vi "Fetch Measurement.vi"(8 "error in (no error)":errorcluster, 9 "Timeout (10000 ms)":u32=10000, 11 "VISA resource name":refnum<visa-resource-name>) -> (0 "error out":errorcluster, 1 "End of Data?":bool, 2 "Measurements":dbl[](array[numeric]), 3 "VISA resource name out":refnum<visa-resource-name>)   [LabVIEW 2020, in "Agilent 34401.lvlib"]
doc: "Fetches the measurement according to the instrument model, trigger source, and math configuration.\n\n<B>Note:</B>\n\nThis VI does not check the instrument status. Typically, you call this VI only in a sequence of calls to other low-level instrument driver VIs. The sequence performs one operation. You use the low-level VIs to optimize one or more aspects of interaction with the instrument. If you want to check the instrument status, call the <B>Error Query VI</B> at the conclusion of the sequence."
uses:
  Agilent 34401.lvlib
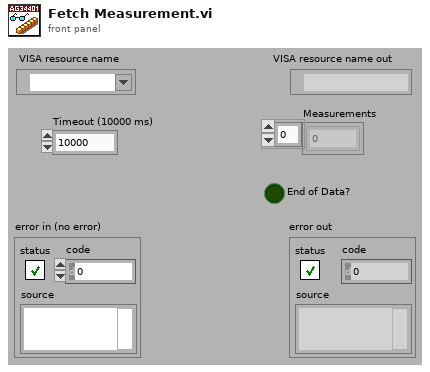
[diagram p1: front panel]
types:
  T1 = typedef "Agilent 34401.lvlib/Extended User Data.ctl" = cluster{"Trigger Source":u16, "Math Storage":u16, "Agilent Model":i32}
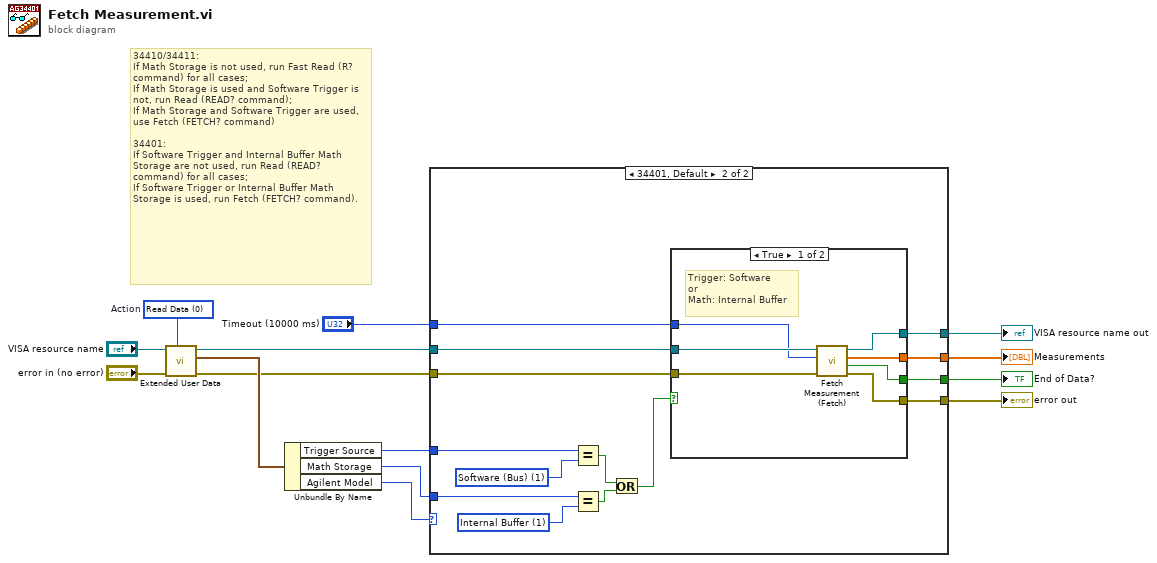
[diagram p0: block diagram]
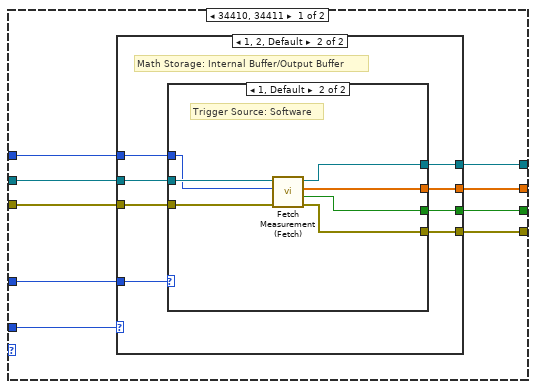
[diagram p2: hidden frame]
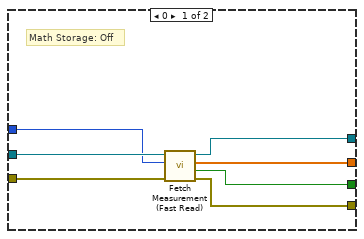
[diagram p3: hidden frame]
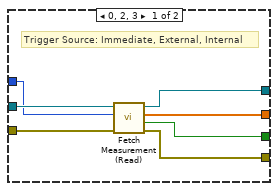
[diagram p4: hidden frame]
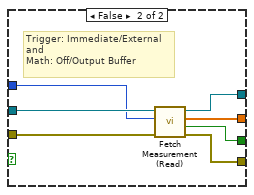
[diagram p5: hidden frame]
diagram:
  w12 = u16 0 items=["Read Data", "Write Data", "Dispose of Data"]  # Action
  # "34410/34411:\nIf Math Storage is not used, run Fast Read (R? command) for all cases;\nIf Math Storage is used and Software Trigger is not, run Read (READ? command);\nIf Math Storage and Software Trigger are used, use Fetch (FETCH? command)\n\n34401:\nIf Software Trigger and Internal Buffer Math Storage are not used, run Read (READ? command) for all cases;\nIf Software Trigger or Internal Buffer Math Storage is used, run Fetch (FETCH? command)."
  n1 = call "Extended User Data.vi"("Action (0: Read Data)"=w12, "Error In (no error)"="error in (no error)", "VISA resource name in"="VISA resource name") -> ("Error Out"=w6:errorcluster, "User Data Out"=w11:T1, "VISA resource name out"=w5:refnum<visa-resource-name>)  [unwired: 6 in]
  n2 = Unbundle By Name(w11) -> ("Trigger Source"=w10:u16, "Math Storage"=w9:u16, "Agilent Model"=w8:i32)
  n3 = case shown="34401, Default" w8 {
    tunnel: w9 -> [w20 w64]
    tunnel: w10 -> [w15 w63]
    tunnel: "Timeout (10000 ms)" -> [w23 w60]
    tunnel: w6 -> [w21 w62]
    tunnel: w5 -> [w22 w61]
    tunnel: [w18 w57] -> w4
    tunnel: [w16 w58] -> w3
    tunnel: [w17 w59] -> w2
    tunnel: [w19 w56] -> w1
    frame 34410, 34411 {
      n4 = case shown="1, 2, Default" w20 {
        tunnel: w23 -> [w28 w35]
        tunnel: w22 -> [w30 w36]
        tunnel: w21 -> [w29 w37]
        tunnel: [w27 w34] -> w19
        tunnel: [w26 w33] -> w18
        tunnel: [w25 w32] -> w17
        tunnel: [w24 w31] -> w16
        tunnel: w15 -> [_ w38]
        frame 0 {
          # "Math Storage: Off"
          n5 = call "Fetch Measurement (Fast Read).vi"("error in (no error)"=w29, "Timeout (10000 ms)"=w28, "VISA resource name"=w30) -> ("error out"=w25:errorcluster, "End of Data?"=w24:bool, "Measurements"=w26:dbl[], "VISA resource name out"=w27:refnum<visa-resource-name>)  [unwired: 5 in]
        }
        frame 1, 2, Default {
          # "Math Storage: Internal Buffer/Output Buffer"
          n6 = case shown="1, Default" w38 {
            tunnel: w37 -> [w44 w52]
            tunnel: w36 -> [w45 w51]
            tunnel: w35 -> [w43 w50]
            tunnel: [w42 w49] -> w34
            tunnel: [w41 w48] -> w33
            tunnel: [w40 w47] -> w32
            tunnel: [w39 w46] -> w31
            frame 0, 2, 3 {
              # "Trigger Source: Immediate, External, Internal"
              n7 = call "Fetch Measurement (Read).vi"("error in (no error)"=w44, "Timeout (10000 ms)"=w43, "VISA resource name"=w45) -> ("error out"=w40:errorcluster, "End of Data?"=w39:bool, "Measurements"=w41:dbl[], "VISA resource name out"=w42:refnum<visa-resource-name>)  [unwired: 5 in]
            }
            frame 1, Default {
              # "Trigger Source: Software"
              n8 = call "Fetch Measurement (Fetch).vi"("error in (no error)"=w52, "Timeout (10000 ms)"=w50, "VISA resource name"=w51) -> ("error out"=w47:errorcluster, "End of Data?"=w46:bool, "Measurements"=w48:dbl[], "VISA resource name out"=w49:refnum<visa-resource-name>)  [unwired: 5 in]
            }
          }
        }
      }
    }
    frame 34401, Default {
      w55 = u16 1 items=["Immediate", "Software (Bus)", "External", "Internal"] ("Trigger Source")
      w54 = u16 1 items=["Off", "Internal Buffer", "Output Buffer"] ("Math Storage")
      n9 = Equal?(x=w63, y=w55) -> (x = y?=w65:bool)
      n10 = Equal?(x=w64, y=w54) -> (x = y?=w66:bool)
      n11 = Or(x=w65, y=w66) -> (x .or. y?=w53:bool)
      n12 = case shown="True" w53 {
        tunnel: w62 -> [w73 w80]
        tunnel: w61 -> [w72 w79]
        tunnel: w60 -> [w71 w74]
        tunnel: [w67 w78] -> w56
        tunnel: [w70 w77] -> w59
        tunnel: [w68 w76] -> w57
        tunnel: [w69 w75] -> w58
        frame True {
          # "Trigger: Software\nor \nMath: Internal Buffer"
          n13 = call "Fetch Measurement (Fetch).vi"("error in (no error)"=w73, "Timeout (10000 ms)"=w71, "VISA resource name"=w72) -> ("error out"=w70:errorcluster, "End of Data?"=w69:bool, "Measurements"=w68:dbl[], "VISA resource name out"=w67:refnum<visa-resource-name>)  [unwired: 5 in]
        }
        frame False {
          # "Trigger: Immediate/External\nand\nMath: Off/Output Buffer"
          n14 = call "Fetch Measurement (Read).vi"("error in (no error)"=w80, "Timeout (10000 ms)"=w74, "VISA resource name"=w79) -> ("error out"=w77:errorcluster, "End of Data?"=w75:bool, "Measurements"=w76:dbl[], "VISA resource name out"=w78:refnum<visa-resource-name>)  [unwired: 5 in]
        }
      }
    }
  }
  "error out" <- w2
  "VISA resource name out" <- w1
  "Measurements" <- w4
  "End of Data?" <- w3
